vi "电脑二运行状态信号转换.vi"() -> ()   [LabVIEW 2017]
panel:
  out "电脑二字符检测运行状态out":bool
  in  "电脑二字符检测运行状态":bool
  out "电脑二压力表检测运行状态out":bool
  in  "电脑二压力表检测运行状态":bool
  out "电脑二压力表打印运行状态out":bool
  in  "电脑二压力表打印运行状态":bool
  out "电脑二封口检测运行状态out":bool
  in  "电脑二封口检测运行状态":bool
  out "电脑二标签检测运行状态out":bool
  in  "电脑二标签检测运行状态":bool
  out "电脑二标签打印运行状态out":bool
  in  "电脑二标签打印运行状态":bool
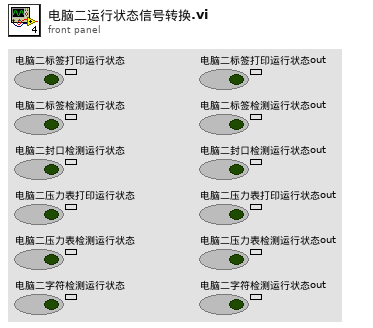
[diagram p1: front panel]
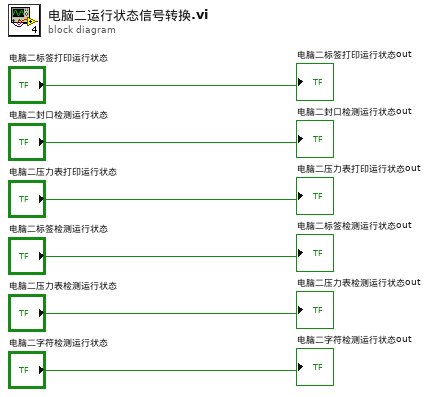
[diagram p0: block diagram]
diagram:
  "电脑二标签打印运行状态out" <- "电脑二标签打印运行状态"
  "电脑二标签检测运行状态out" <- "电脑二标签检测运行状态"
  "电脑二封口检测运行状态out" <- "电脑二封口检测运行状态"
  "电脑二压力表打印运行状态out" <- "电脑二压力表打印运行状态"
  "电脑二压力表检测运行状态out" <- "电脑二压力表检测运行状态"
  "电脑二字符检测运行状态out" <- "电脑二字符检测运行状态"
